vi "Initialize.vi"(8 "error in (no error)":errorcluster, 10 "Laser Configuration":T1, 11 "LQ Laser Quantum in":refnum<class "LQ Laser.lvclass">) -> (0 "error out":errorcluster, 3 "LQ Laser Quantum out":refnum<class "LQ Laser.lvclass">)   [LabVIEW 2023, in "LQ Laser.lvlib" / "LQ Laser.lvclass"]
uses:
  LQ Laser.lvclass
  Resources/Type Defs/Laser Configuration.ctl
  LQ Laser.lvclass/LQ Laser.ctl
  <vilib>/Instr/_visa.llb/VISA Configure Serial Port (Instr).vi
  Laser/Laser.lvclass
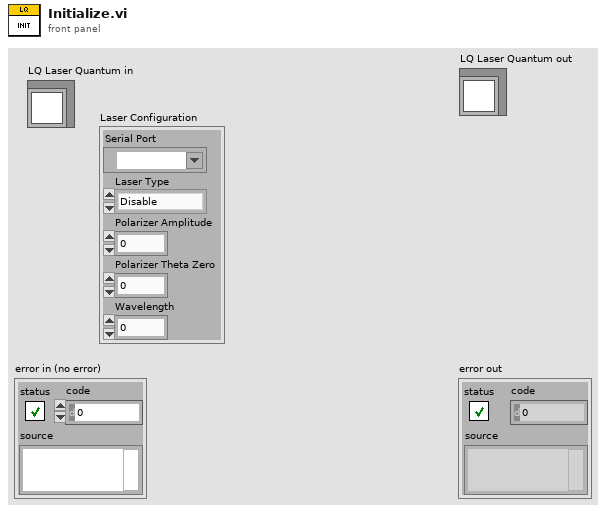
[diagram p1: front panel]
types:
  T1 = typedef "Laser Configuration.ctl" = cluster{"Serial Port":refnum<visa-resource-name>, "Laser Type":enum16{"Disable", "Laser Quantum", "Coherent OBIS", "PRM1-Z8", "Coherent HOPS"}, "Polarizer Amplitude":dbl, "Polarizer Theta Zero":dbl, "Wavelength":u16}
  T2 = enum16{"Disable", "Laser Quantum", "Coherent OBIS", "PRM1-Z8", "Coherent HOPS"}
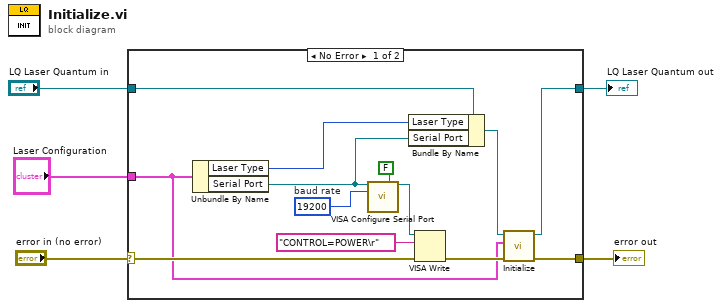
[diagram p0: block diagram]
diagram:
  n1 = case shown="No Error" "error in (no error)" {
    selector: "error in (no error)" -> [w18 w19]
    tunnel: [w7 w19] -> w3
    tunnel: "Laser Configuration" -> [w8 _]
    tunnel: "LQ Laser Quantum in" -> [w13 w20]
    tunnel: [w6 w20] -> w2
    frame No Error {
      w15 = u32 19200  # baud rate
      n2 = Unbundle By Name(w8) -> ("Laser Type"=w11:T2, "Serial Port"=w12:refnum<visa-resource-name>)
      n3 = call-poly "VISA Configure Serial Port"("VISA resource name"=w12, "Enable Termination\nChar (T)"=FALSE ("Enable Termination\nChar (T)"), "baud rate (9600)"=w15) -> ("VISA resource name out"=w17:refnum<visa-resource-name>)  [unwired: 11 in, 1 out]
      n4 = Bundle By Name(cluster=w13, "Laser Type"=w11, "Serial Port"=w12) -> (w9:refnum<class "LQ Laser.lvclass">)
      n5 = VISA Write(VISA resource name=w17, write buffer="CONTROL=POWER\r", error in (no error)=w18) -> (error out=w10:errorcluster)  [unwired: 2 out]
      n6 = call-parent "Initialize.vi"("error in (no error)"=w10, "Laser Configuration"=w8, "Laser in"=w9) -> ("error out"=w7:errorcluster, "Laser out"=w6:refnum<class "LQ Laser.lvclass">)  [unwired: 7 in]
    }
    frame Error {
    }
  }
  "error out" <- w3
  "LQ Laser Quantum out" <- w2
